vi "Network-Find Next Available EndPoint.vi"() -> (4 "address":string, 6 "port":u16, 15 "error out":errorcluster)   [LabVIEW 2020]
panel:
  in  "Excludes":string[](array[string])
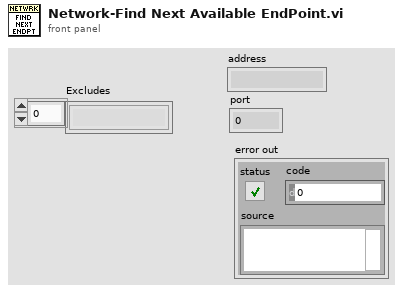
[diagram p1: front panel]
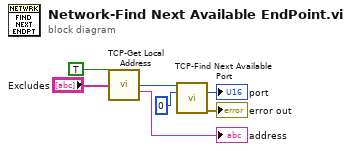
[diagram p0: block diagram]
diagram:
  n1 = call "TCP-Get Local Address.vi"("LAN first"=TRUE, "Excludes"="Excludes") -> ("net address"=w5:u32, "address"=→"address":string)  [unwired: 12 in]
  n2 = call "TCP-Find Next Available Port.vi"("net address"=w5, "start"=u16 0) -> ("port"=→"port":u16, "error out"=→"error out":errorcluster)  [unwired: 12 in]
